vi "Spreadsheet to array.vi"(6 "start of read offset (chars.:0)":i32, 7 "max characters/row  (no limit:0)":i32, 9 "number of rows (all:-1)":i32=-1, 10 "format (%d)":string="%d", 11 "file path (dialog if empty) in":path) -> (1 "mark after read (chars.)":i32, 3 "new file path (Not A Path if cancelled)":path, 4 "EOF?":bool)   [LabVIEW 2013]
panel:
  out "array":u16[](array[numeric])
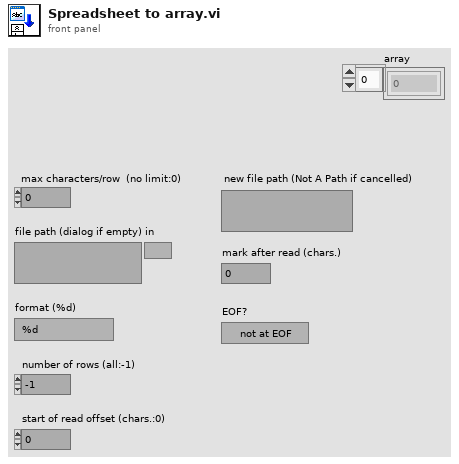
[diagram p1: front panel]
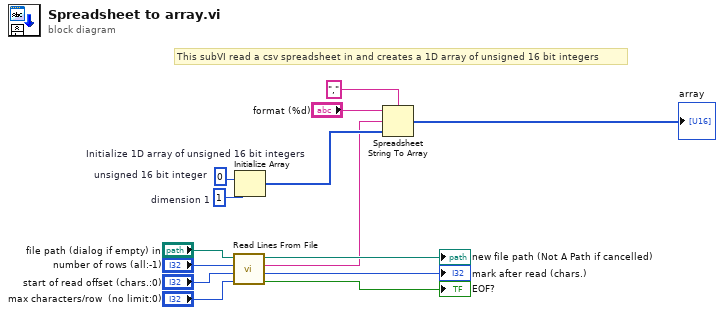
[diagram p0: block diagram]
diagram:
  w12 = u16 0  # unsigned 16 bit integer
  w13 = 1  # dimension 1
  # "This subVI read a csv spreadsheet in and creates a 1D array of unsigned 16 bit integers"
  n1 = call <vilib>:"Read Lines From File.vi"("file path (dialog if empty)"="file path (dialog if empty) in", "number of lines (all:-1)"="number of rows (all:-1)", "start of read offset (chars.:0)"="start of read offset (chars.:0)", "[max characters per line]  (no limit:0)"="max characters/row  (no limit:0)") -> ("new file path (Not A Path if cancelled)"=→"new file path (Not A Path if cancelled)":path, "line string"=w2:string, "mark after read (chars.)"=→"mark after read (chars.)":i32, "EOF?"=→"EOF?":bool)  [unwired: 2 in]
  n2 = Initialize Array "Initialize 1D array of unsigned 16 bit integers"(w12, w13) -> (w14:u16[])
  n3 = Spreadsheet String To Array(delimiter (Tab)=",", format string="format (%d)", spreadsheet string=w2, array type (2D Dbl)=w14) -> (array=→"array":u16[])
